vi "KeyboardCalls.vi"(11 "Cluster":T2) -> (1 "Extras":enum16{"Nix", "clear"}(ring), 3 "string":string)   [LabVIEW 2020]
uses:
  <vilib>/event_ctls.llb/eventvkey.ctl
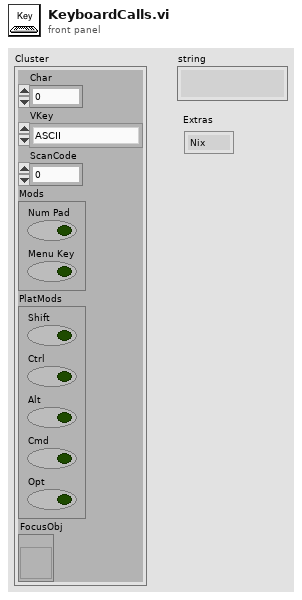
[diagram p1: front panel]
types:
  T1 = typedef "eventvkey.ctl" = enum16{"ASCII", "Enter", "Return", "Shift", "Ctrl", "Alt", "Cmd", "Opt", "Caps", "NumLock", "Clear", "Break", "Up", "Down", "Left", "Right", "Insert", "Delete", "Home", "End", "PageUp", "PageDown", "Escape", "Help", "Pause", "ScrollLock", "F1", "F2", "F3", "F4", "F5", "F6", "F7", "F8", "F9", "F10", "F11", "F12", "F13", "F14", "F15", "F16", "F17", "F18", "F19", "F20", "F21", "F22", "F23", "F24", "Play", "VolumeUp", "VolumeDown", "Mute", "Two Byte Char"}
  T2 = cluster{"Char":i16, "VKey":T1, "ScanCode":i16, "Mods":cluster{"Num Pad":bool, "Menu Key":bool}, "PlatMods":cluster{"Shift":bool, "Ctrl":bool, "Alt":bool, "Cmd":bool, "Opt":bool}, "FocusObj":refnum<vi>}
  T3 = cluster{"Shift":bool, "Ctrl":bool, "Alt":bool, "Cmd":bool, "Opt":bool}
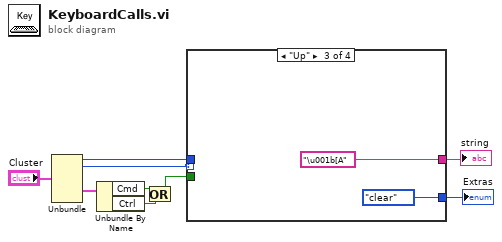
[diagram p0: block diagram]
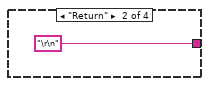
[diagram p3: hidden frame]
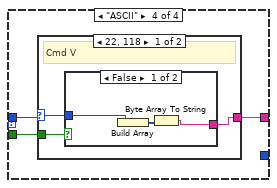
[diagram p4: hidden frame]
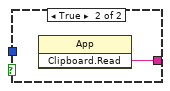
[diagram p5: hidden frame]
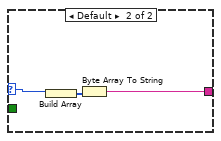
[diagram p6: hidden frame]
diagram:
  n1 = Unbundle("Cluster") -> ("Char"=w7:i16, "VKey"=w6:T1, "PlatMods"=w5:T3)  [unwired: 3 out]
  n2 = Unbundle By Name(w5) -> ("Cmd"=w4:bool, "Ctrl"=w3:bool)
  n3 = Or(x=w4, y=w3) -> (x .or. y?=w2:bool)
  n4 = case shown="\"Up\"" w6 {
    tunnel: [_ "\r\n" ("string") "\u001b[A" ("string") w15] -> w9
    tunnel: w7 -> [_ _ _ w14]
    tunnel: w2 -> [_ _ _ w13]
    tunnel: [_ _ enum16{"Nix", "clear"}."clear" ("Clear line?") _] -> w1
    frame Default {
    }
    frame "Return" {
    }
    frame "Up" {
    }
    frame "ASCII" {
      n5 = case shown="22, 118" w14 {
        selector: w14 -> [w16 w23]
        tunnel: [w18 w25] -> w15
        tunnel: w13 -> [w17 _]
        frame 22, 118 {
          # "Cmd V"
          n6 = case shown="False" w17 {
            tunnel: [w19 w22] -> w18
            tunnel: w16 -> [w20 _]
            frame False {
              n7 = Build Array(w20) -> (w21:i16[])
              n8 = Byte Array To String(unsigned byte array=w21) -> (string=w19:string)
            }
            frame True {
              n9 = invoke class="App" method="Clipboard.Read"() -> ("Read Clipbrd"=w22:string)  [unwired: 3 in, 2 out]
            }
          }
        }
        frame Default {
          n10 = Build Array(w23) -> (w24:i16[])
          n11 = Byte Array To String(unsigned byte array=w24) -> (string=w25:string)
        }
      }
    }
  }
  "string" <- w9
  "Extras" <- w1
